vi "medicaoIXV.vi"() -> ()   [LabVIEW 2012]
uses:
  <vilib>/Utility/file.llb/Write To Spreadsheet File (string).vi
  <vilib>/Utility/file.llb/Write To Spreadsheet File (DBL).vi
  <instrlib>/Agilent 6XXX Series/Agilent 6XXX Series.lvlib
  <vilib>/Analysis/NI_AALBase.lvlib
panel:
  out "current time":timestamp
  out "stopLoopMedicoes":bool caption="Parar Medição"
  out "desvio":dbl format="%0.2f"
  out "reset graph":bool=TRUE
  out "tabela":dbl[][](array[numeric])
  in  "Tab Control":enum32{"Entrada de dados", "Saída de dados"}(tab)
  in  "Irradiância":dbl caption="Irradiância(W/m²)"
  in  "nCurvas":i64=1 caption="Nº de curvas" min=1
  in  "T.J":dbl caption="Tensão\ndo joelho" step=0.1
  in  "p.a.j":dbl caption="Pontos antes\ndo joelho"
  in  "nMedições":i16=1 caption="N° medições por ponto" min=1
  in  "area":dbl caption="Área da célula(cm²)"
  in  "Tipo":string caption="Tipo da célula"
  in  "Formato":u16(ring) items=[".txt", ".csv"]
  out "ON/OFF1":bool caption="ON/OFF"
  in  "p.d.j":dbl caption="Pontos depois\ndo joelho"
  in  "T.M":dbl caption="Tensão máxima" step=0.1
  in  "Nome da célula":string
  in  "Local":path
  in  "Delay(ms)":dbl
  in  "Start":bool
  in  "temperatura":dbl caption="Temperatura da célula"
  out "tempo de medição":dbl
  in  "stopProgram":bool caption="Parar Programa"
  out "Imp":dbl caption="Imp(A)"
  out "Vmp":dbl caption="Vmp(V)"
  out "Pmp":dbl caption="Pmp(W)"
  out "Icc (A)":dbl
  out "Vca (V)":dbl
  in  "Print Screen":bool
  out "IXV":cluster{"Y":dbl[], "Y":dbl[]}[](graph)
  out "output voltage":dbl
  out "vAtual":dbl caption="Tensao Atual (V)"
  out "aAtual":dbl caption="Corrente Atual\n(A)"
  out "Ponto Atual":i32
  out "tabela":dbl[][](array[numeric]) caption="TABELA DE DADOS\nTensão(Fonte)      Pontos             Tensao           Corrente" format="%0.8f"
  in  "stop":bool caption="Parar Medição"
  out "ON/OFF2":bool caption="ON/OFF"
  out "eficiencia":dbl caption="Eficiencia(%)"
  out "FF":dbl
  in  "CorrenteGraph":dbl
  in  "TensaoGraph":dbl
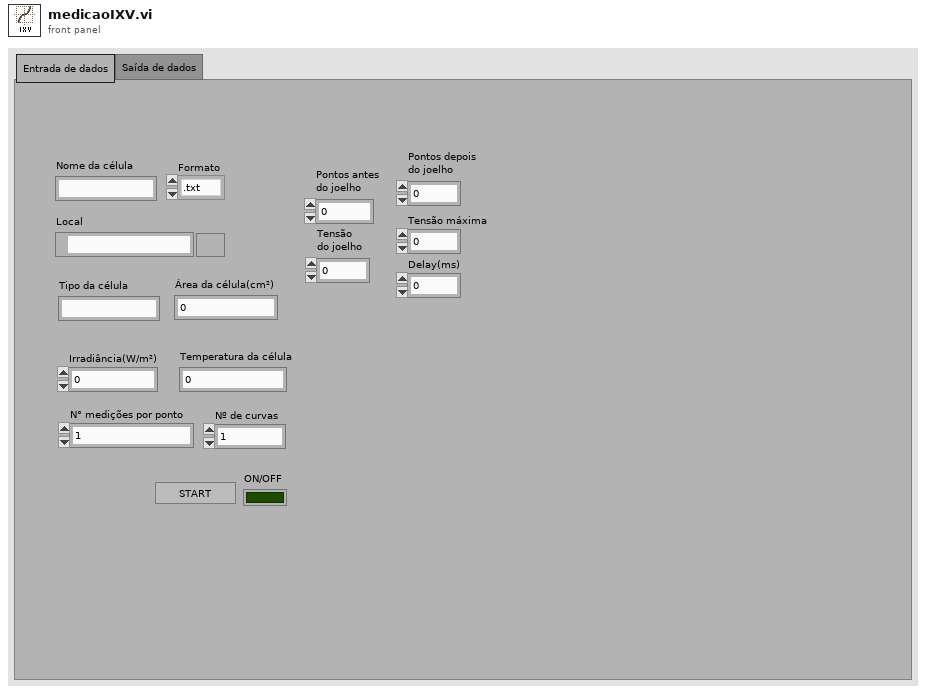
[diagram p1: front panel]
types:
  T1 = typedef "imagedata.ctl" = cluster{"image type":i32, "image depth":i32, "image":u8[], "mask":u8[], "colors":u32[], "Rectangle":cluster{"left":i16, "top":i16, "right":i16, "bottom":i16}}
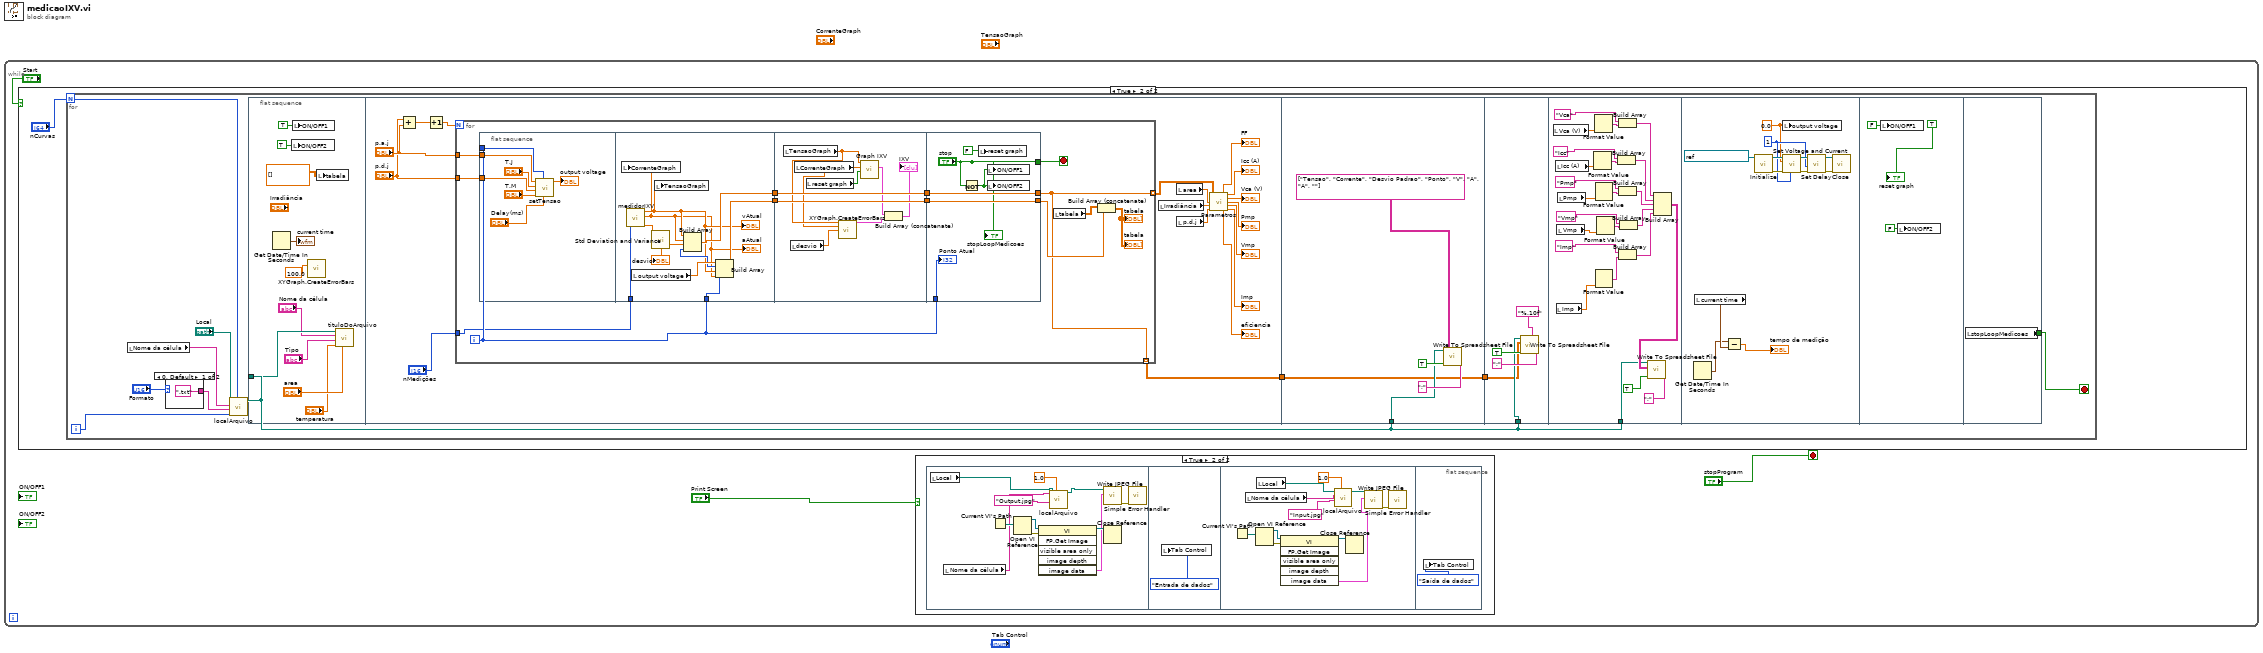
[diagram p0: block diagram]
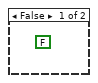
[diagram p3: hidden frame]
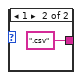
[diagram p4: hidden frame]
diagram:
  n1 = while {
    stop <- "stopProgram" stop-if-true
    n2 = case shown="True" "Start" {
      frame False {
        (unwired) FALSE
      }
      frame True {
        n3 = for {
          N: "nCurvas" -> [w31]
          i -> [w30]
          stop <- w29 stop-if-true
          n4 = local read "Nome da célula"() -> (w34:string)
          n5 = case shown="0, Default" "Formato" {
            tunnel: [".txt" ".csv"] -> w33
            frame 0, Default {
            }
            frame 1 {
            }
          }
          n6 = call "localArquivo.vi"("quantidadeDeArquivos"=w31, "numeroDoArquivo"=w30, "extensão"=w33, "Nome do arquivo"=w34, "Local"="Local") -> ("Path"=w32:path)  [unwired: 6 in]
          n7 = flat-sequence {
            tunnel: w32 -> [w50]
            tunnel: [w63] -> w38
            tunnel: w32 -> [w114]
            tunnel: [w113] -> w37
            tunnel: w38 -> [w113]
            tunnel: w32 -> [w118]
            tunnel: w37 -> [w117]
            tunnel: w32 -> [w122]
            tunnel: [w161] -> w29
            frame #0 {
              n8 = Get Date/Time In Seconds() -> (seconds since 1Jan1904=→"current time":timestamp)
              n9 = local write "ON/OFF2"(TRUE ("ON/OFF2")) -> ()
              n10 = local write "ON/OFF1"(TRUE ("ON/OFF")) -> ()
              n11 = call "XYGraph.CreateErrorBars.vi"("yTemp"=100.0) -> ()  [unwired: 14 in, 1 out]
              n12 = local write "tabela"(dbl[][] [] ("array")) -> ()
              n13 = call "tituloDoArquivo.vi"("area"="area", "temperatura"="temperatura", "Tipo"="Tipo", "Nome da célula"="Nome da célula", "file path (dialog if empty)"=w50) -> ()  [unwired: 7 in]
            }
            frame #1 {
              n14 = Add(x="p.d.j", y="p.a.j") -> (x+y=w66:dbl)
              n15 = Increment(x=w66) -> (x+1=w67:dbl)
              n16 = for {
                N: w67 -> [_]
                tunnel: [w68] -> w55 mode=indexing
                tunnel: "p.a.j" -> [w71]
                tunnel: "p.d.j" -> [w70]
                tunnel: "nMedições" -> [w69]
                tunnel: [w68] -> w63 mode=indexing
                i -> [w75]
                stop <- w74 stop-if-true
                n17 = flat-sequence {
                  tunnel: w75 -> [w86]
                  tunnel: w71 -> [w84]
                  tunnel: w70 -> [w83]
                  tunnel: w75 -> [w91]
                  tunnel: [w94] -> w80
                  tunnel: [w96] -> w79
                  tunnel: w69 -> [w93]
                  tunnel: [w105] -> w73
                  tunnel: [w104] -> w72
                  tunnel: w79 -> [w104]
                  tunnel: w80 -> [w105]
                  tunnel: [w110] -> w78
                  tunnel: [w111] -> w68
                  tunnel: w73 -> [w111]
                  tunnel: w72 -> [w110]
                  tunnel: w75 -> [w109]
                  tunnel: ["stop"] -> w74
                  frame #0 {
                    n18 = call "setTensao.vi"("delay(ms)"="Delay(ms)", "Ponto atual"=w86, "T.M"="T.M", "P.D.J"=w83, "T.J"="T.J", "P.A.J"=w84) -> ("output voltage"=→"output voltage":dbl)  [unwired: 5 in]
                  }
                  frame #1 {
                    n19 = call "medidorIXV.vi"("nMedicoes"=w93) -> ("Tensao Atual"=w90:dbl, "Corrente Atual"=w89:dbl, "vetorCorrente"=w92:dbl[])  [unwired: 7 in]
                    "aAtual" <- w89
                    "vAtual" <- w90
                    n20 = local write "CorrenteGraph"(w89) -> ()
                    n21 = local read "output voltage"() -> (w95:dbl)
                    n22 = call <vilib>:"Std Deviation and Variance.vi"("X"=w92) -> ("standard deviation"=w88:dbl)  [unwired: 1 in, 2 out]
                    "desvio" <- w88
                    n23 = local write "TensaoGraph"(w90) -> ()
                    n24 = Build Array(w90, w89, w88, w91) -> (w94:dbl[])
                    n25 = Build Array(w95, w91, w90, w89) -> (w96:dbl[])
                  }
                  frame #2 {
                    n26 = local read "TensaoGraph"() -> (w99:dbl)
                    n27 = local read "desvio"() -> (w97:dbl)
                    n28 = local read "CorrenteGraph"() -> (w98:dbl)
                    n29 = local read "reset graph"() -> (w103:bool)
                    n30 = call "XYGraph.CreateErrorBars.vi"("xTemp"=w99, "yTemp"=w98, "errorTemp"=w97) -> ("error bar plot"=w100:cluster{dbl[], dbl[]})  [unwired: 12 in]
                    n31 = call "Graph IXV"("Reset"=w103, "Y Input"=w98, "X Input"=w99) -> ("XY Graph"=w102:cluster{"Y":dbl[], "Y":dbl[]}[])  [unwired: 2 in, 6 out]
                    n32 = Build Array (concatenate)(w102, w100) -> (→"IXV":cluster{"Y":dbl[], "Y":dbl[]}[])
                  }
                  frame #3 {
                    n33 = Not(x="stop") -> (.not. x?=w107:bool)
                    n34 = local write "reset graph"(FALSE) -> ()
                    n35 = local write "ON/OFF1"(w107) -> ()
                    n36 = local write "ON/OFF2"(w107) -> ()
                    "Ponto Atual" <- w109
                    "stopLoopMedicoes" <- "stop"
                  }
                }
                n37 = local read "tabela"() -> (w77:dbl[][])
                n38 = Build Array (concatenate)(w77, w78) -> (→"tabela" →"tabela":dbl[][])
              }
              n39 = local read "Irradiância"() -> (w53:dbl)
              n40 = local read "area"() -> (w54:dbl)
              n41 = local read "p.d.j"() -> (w56:dbl)
              n42 = call "Parametros.vi"("VetorDeDados"=w55, "area"=w54, "irradiancia"=w53, "pontos"=w56) -> ("FF"=→"FF":dbl, "Icc"=→"Icc (A)":dbl, "Vca"=→"Vca (V)":dbl, "Pmp"=→"Pmp":dbl, "Vmp"=→"Vmp":dbl, "eficiencia"=→"eficiencia":dbl, "Imp"=→"Imp":dbl)  [unwired: 5 in]
            }
            frame #2 {
              n43 = call-poly <vilib>:"Write To Spreadsheet File.vi"("delimiter (\\t)"=";" ("delimiter (\\t)"), "append to file? (new file:F)"=TRUE, "2D data"=string[][] [["Tensao", "Corrente", "Desvio Padrao", "Ponto"], ["V", "A", "A", ""]], "file path (dialog if empty)"=w114) -> ()  [unwired: 4 in, 1 out]
            }
            frame #3 {
              n44 = call-poly <vilib>:"Write To Spreadsheet File.vi"("delimiter (\\t)"=";" ("delimiter (\\t)"), "format (%.3f)"="%.10f", "append to file? (new file:F)"=TRUE, "2D data"=w117, "file path (dialog if empty)"=w118) -> ()  [unwired: 3 in, 1 out]
            }
            frame #4 {
              n45 = local read "Vca (V)"() -> (w124:dbl)
              n46 = local read "Icc (A)"() -> (w134:dbl)
              n47 = local read "Imp"() -> (w137:dbl)
              n48 = local read "Vmp"() -> (w136:dbl)
              n49 = local read "Pmp"() -> (w135:dbl)
              n50 = Format Value(value (0)=w134) -> (output string=w127:string)  [unwired: 2 in]
              n51 = Format Value(value (0)=w124) -> (output string=w125:string)  [unwired: 2 in]
              n52 = Format Value(value (0)=w135) -> (output string=w129:string)  [unwired: 2 in]
              n53 = Format Value(value (0)=w137) -> (output string=w133:string)  [unwired: 2 in]
              n54 = Format Value(value (0)=w136) -> (output string=w131:string)  [unwired: 2 in]
              n55 = Build Array("Icc", w127) -> (w139:string[])
              n56 = Build Array("Vca", w125) -> (w138:string[])
              n57 = Build Array("Pmp", w129) -> (w140:string[])
              n58 = Build Array("Imp", w133) -> (w142:string[])
              n59 = Build Array("Vmp", w131) -> (w141:string[])
              n60 = Build Array(w138, w139, w140, w141, w142) -> (w143:string[][])
              n61 = call-poly <vilib>:"Write To Spreadsheet File.vi"("delimiter (\\t)"=";" ("delimiter (\\t)"), "append to file? (new file:F)"=TRUE, "2D data"=w143, "file path (dialog if empty)"=w122) -> ()  [unwired: 4 in, 1 out]
            }
            frame #5 {
              w149 = 0.0 ("voltage (0 V)")
              w152 = u8 1 ("channel (1)")
              n62 = Get Date/Time In Seconds() -> (seconds since 1Jan1904=w146:timestamp)
              n63 = local read "current time"() -> (w147:timestamp)
              n64 = Subtract(x=w146, y=w147) -> (x-y=→"tempo de medição":dbl)
              n65 = call <instrlib>:"Initialize.vi"("VISA resource name"=refnum<visa-resource-name> "GPIB0::5::INSTR") -> ("error out"=w154:errorcluster, "VISA resource name out"=w153:refnum<visa-resource-name>)  [unwired: 9 in]
              n66 = local write "output voltage"(w149) -> ()
              n67 = call <instrlib>:"Set Voltage and Current.vi"("channel (1)"=w152, "error in (no error)"=w154, "voltage (0 V)"=w149, "VISA resource name"=w153) -> ("error out"=w155:errorcluster, "VISA resource name out"=w156:refnum<visa-resource-name>)  [unwired: 6 in]
              n68 = call <instrlib>:"Set Delay.vi"("error in (no error)"=w155, "channel (1)"=w152, "VISA resource name"=w156) -> ("error out"=w150:errorcluster, "VISA resource name out"=w151:refnum<visa-resource-name>)  [unwired: 7 in]
              n69 = call <instrlib>:"Close.vi"("error in (no error)"=w150, "VISA resource name"=w151) -> ()  [unwired: 9 in, 1 out]
            }
            frame #6 {
              n70 = local write "ON/OFF1"(FALSE) -> ()
              n71 = local write "ON/OFF2"(FALSE ("ON/OFF")) -> ()
              "reset graph" <- TRUE
            }
            frame #7 {
              n72 = local read "stopLoopMedicoes"() -> (w161:bool)
            }
          }
        }
      }
    }
    n73 = case shown="True" "Print Screen" {
      frame False {
      }
      frame True {
        n74 = flat-sequence {
          frame #0 {
            n75 = local read "Local"() -> (w7:path)
            n76 = local read "Nome da célula"() -> (w5:string)
            n77 = Current VI's Path() -> (path=w12:path)
            n78 = Open VI Reference(vi path=w12) -> (vi reference=w13:refnum<vi>, error out=w14:errorcluster)  [unwired: 5 in]
            n79 = invoke class="VI" method="FP.Get Image"(reference=w13, error in=w14) -> (reference out=w11:refnum<vi>, "image data"=w10:T1)  [unwired: 4 in, 4 out]
            n80 = call "localArquivo.vi"("quantidadeDeArquivos"=1.0, "extensão"="Output.jpg", "Nome do arquivo"=w5, "Local"=w7) -> ("Path"=w4:path)  [unwired: 7 in]
            n81 = call <vilib>:"Write JPEG File.vi"("image data"=w10, "path to JPEG file"=w4) -> ("error out"=w9:errorcluster)  [unwired: 8 in, 1 out]
            n82 = Close Reference(reference=w11) -> ()  [unwired: 1 in, 1 out]
            n83 = call <vilib>:"Simple Error Handler.vi"("error in (no error)"=w9) -> ()  [unwired: 4 in, 5 out]
          }
          frame #1 {
            n84 = local write "Tab Control"(enum32{"Entrada de dados", "Saída de dados"}."Entrada de dados" ("Tab Control")) -> ()
          }
          frame #2 {
            n85 = Current VI's Path() -> (path=w25:path)
            n86 = local read "Nome da célula"() -> (w19:string)
            n87 = Open VI Reference(vi path=w25) -> (vi reference=w24:refnum<vi>, error out=w23:errorcluster)  [unwired: 5 in]
            n88 = local read "Local"() -> (w18:path)
            n89 = invoke class="VI" method="FP.Get Image"(reference=w24, error in=w23) -> (reference out=w26:refnum<vi>, "image data"=w21:T1)  [unwired: 4 in, 4 out]
            n90 = call "localArquivo.vi"("quantidadeDeArquivos"=1.0, "extensão"="Input.jpg", "Nome do arquivo"=w19, "Local"=w18) -> ("Path"=w17:path)  [unwired: 7 in]
            n91 = Close Reference(reference=w26) -> ()  [unwired: 1 in, 1 out]
            n92 = call <vilib>:"Write JPEG File.vi"("image data"=w21, "path to JPEG file"=w17) -> ("error out"=w22:errorcluster)  [unwired: 8 in, 1 out]
            n93 = call <vilib>:"Simple Error Handler.vi"("error in (no error)"=w22) -> ()  [unwired: 4 in, 5 out]
          }
          frame #3 {
            n94 = local write "Tab Control"(enum32{"Entrada de dados", "Saída de dados"}."Saída de dados" ("Tab Control")) -> ()
          }
        }
      }
    }
  }
